vi "Read Action command queues.vi"(11 "Communication in":refnum<class "Communication.lvclass">) -> (2 "Action command queues out":refnum<queue>[](array[refnum]))   [LabVIEW 2021, in "Communication.lvclass"]
doc: "MIT Licence\nCopyright (c) 2024 David Grollier"
uses:
  Communication.lvclass
  Game Componants/Game Board/Action Command.ctl
  Communication.lvclass/Communication.ctl
  Game Componants/Game Board/Game Board.lvclass
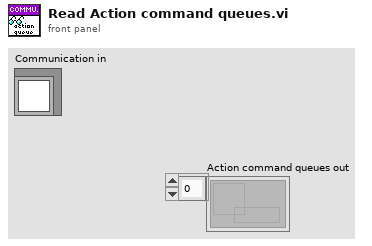
[diagram p1: front panel]
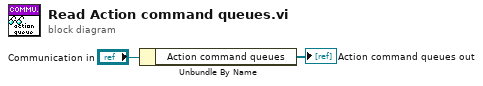
[diagram p0: block diagram]
diagram:
  n1 = Unbundle By Name("Communication in") -> ("Action command queues"=→"Action command queues out":refnum<queue>[])
